vi "Configure_DMM.vi"(8 "error in (no error)":errorcluster, 10 "DMM_Configuration":T1={"Range"=10.0, "Measurement Type"=enum."DC Volts", "Resolution in Digits"=enum."5 1/2", "pin or relay names"=""} {"Range" format="%.2f"}, 11 "DMM_Base in":refnum<class "DMM_Base.lvclass">) -> (0 "error out":errorcluster, 3 "DMM_Base out":refnum<class "DMM_Base.lvclass">)   [LabVIEW 2020, in "DMM_Base.lvclass"]
doc: "The API configures the DMM instrument connected to the given pin in <b>DMM_Configuration</b>"
uses:
  DMM_Base.lvclass
  Typedef/DMM_Configuration.ctl
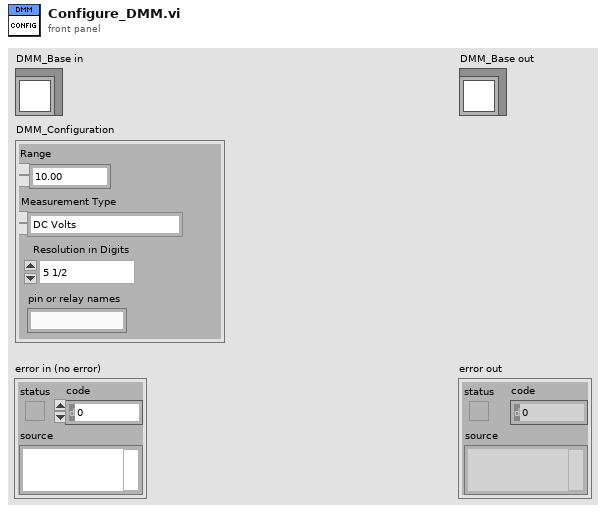
[diagram p1: front panel]
types:
  T1 = typedef "DMM_Base.lvclass/DMM_Configuration.ctl" = cluster{"Range":dbl, "Measurement Type":enum32{"DC Volts", "AC Volts", "DC Current", "AC Current", "2-wire Resistance", "4-wire Resistance", "Diode", "Frequency", "Period", "AC Volts DC Coupled", "Capacitance", "Inductance", "Temperature"}, "Resolution in Digits":enum32{"3 1/2", "4 1/2", "5 1/2", "6 1/2", "7 1/2"}, "pin or relay names":string}
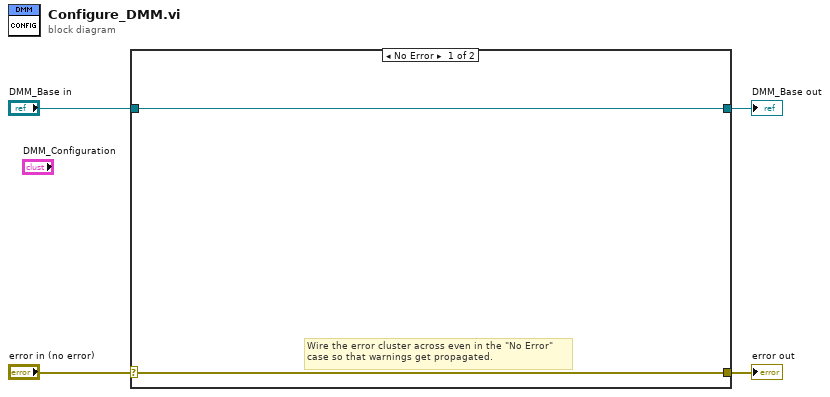
[diagram p0: block diagram]
diagram:
  n1 = case shown="No Error" "error in (no error)" {
    selector: "error in (no error)" -> [w5 w8]
    tunnel: [w5 w8] -> w3
    tunnel: [w6 w7] -> w1
    tunnel: "DMM_Base in" -> [w6 w7]
    frame No Error {
      # "Wire the error cluster across even in the \"No Error\"\ncase so that warnings get propagated."
    }
    frame Error {
    }
  }
  "error out" <- w3
  "DMM_Base out" <- w1
